vi "ForwardForInch.vi"(8 "error in":errorcluster, 11 "Distance":dbl) -> (0 "error out":errorcluster)   [LabVIEW 2016]
uses:
  Robot Global Data.vi
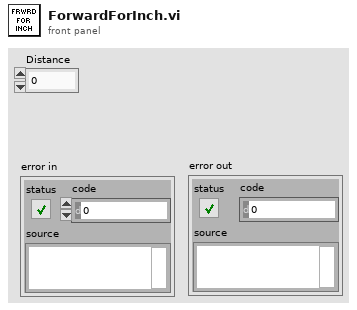
[diagram p1: front panel]
types:
  T1 = cluster{"Lower X":dbl, "Lower Y":dbl, "Upper X":dbl, "Upper Y":dbl}
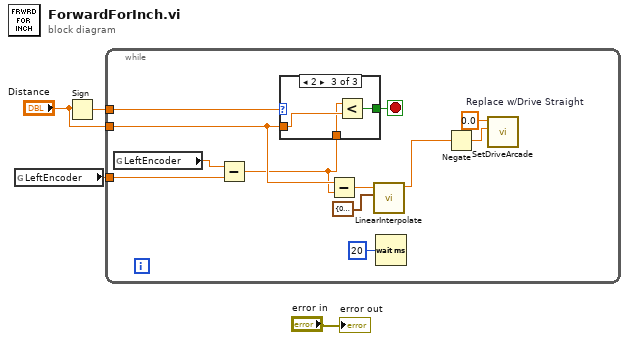
[diagram p0: block diagram]
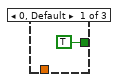
[diagram p2: hidden frame]
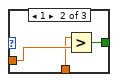
[diagram p3: hidden frame]
diagram:
  n1 = global read "Robot Global Data.vi" "LeftEncoder"() -> (w2:dbl)
  n2 = Sign(1:"Distance") -> (0:w4:dbl)
  n3 = while {
    tunnel: w4 -> [w15]
    tunnel: "Distance" -> [w10]
    tunnel: w2 -> [w13]
    stop <- w14 stop-if-true
    w11 = 0.0  # Replace w/Drive Straight
    n4 = global read "Robot Global Data.vi" "LeftEncoder"() -> (w12:dbl)
    n5 = Subtract(x=w12, y=w13) -> (x-y=w9:dbl)
    n6 = case shown="2" w15 {
      tunnel: [TRUE w20 w23] -> w14
      tunnel: w10 -> [_ w19 w22]
      tunnel: w9 -> [_ w18 w21]
      frame 0, Default {
      }
      frame 1 {
        n7 = Greater?(x=w18, y=w19) -> (0:w20:bool)
      }
      frame 2 {
        n8 = Less?(x=w21, y=w22) -> (x < y?=w23:bool)
      }
    }
    n9 = Subtract(x=w10, y=w9) -> (x-y=w8:dbl)
    n10 = call "LinearInterpolate.vi"("Config"=T1 {"Lower X"=0.0, "Lower Y"=0.4, "Upper X"=100.0, "Upper Y"=0.75}, "Value"=w8) -> ("Output"=w7:dbl)  [unwired: 9 in]
    n11 = Wait (ms)(milliseconds to wait=u32 20) -> ()  [unwired: 1 out]
    n12 = Negate(x=w7) -> (-x=w6:dbl)
    n13 = call "SetDriveArcade.vi"("Forward"=w6, "Turn"=w11) -> ()  [unwired: 10 in]
  }
  "error out" <- "error in"
